vi "Byte Buffer.Read (1D I16).vi"(7 "byte order (big-endian)":T1(ring), 8 "error in (no error)":errorcluster, 9 "count":i32, 10 "buffer offset":i32, 11 "buffer in":string) -> (0 "error out":errorcluster, 1 "value":i16[](array[numeric]), 3 "buffer out":string)   [LabVIEW 2016, in "VeriStand Data.lvlib"]
doc: "Reads <B>count</B> elements of data from the provided <B>buffer</B> at location <B>buffer offset</B> in the format of the data type specified. The data endianness can be specified via <B>byte order</B>."
uses:
  VeriStand Data.lvlib
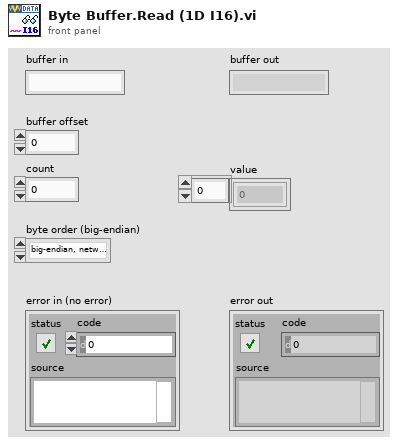
[diagram p1: front panel]
types:
  T1 = enum16{"big-endian, network order", "native, host order", "little-endian"}
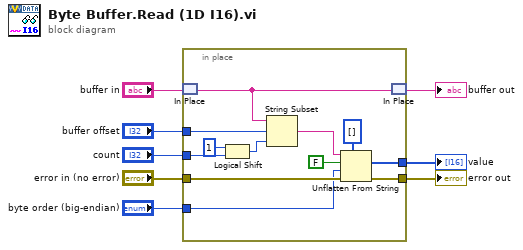
[diagram p0: block diagram]
diagram:
  n1 = in-place {
    in-place-border: "buffer offset" -> [w19]
    in-place-border: "error in (no error)" -> [w17]
    in-place-border: "byte order (big-endian)" -> [w15]
    in-place-border: [w13] -> w4
    in-place-border: [w12] -> w2
    in-place-border: "count" -> [w9]
    n2 = in-place-match #1("buffer in") -> (w20:string)
    n3 = Logical Shift(y=i16 1, x=w9) -> (x << y=w10:i32)
    n4 = String Subset(string=w20, offset (0)=w19, length (rest)=w10) -> (substring=w18:string)
    n5 = Unflatten From String(type=i16[] [], binary string=w18, data includes array or string size? (T)=FALSE, byte order (0:big-endian, network order)=w15, error in (no error)=w17) -> (value=w12:i16[], error out=w13:errorcluster)  [unwired: 1 out]
    n6 = in-place-match #1(w20) -> (→"buffer out":string)
  }
  "value" <- w2
  "error out" <- w4
